vi "CMD_05_SetSendPeriod.vi"(9 "Period, ms":dbl=10.0 min=10.0 max=10000.0, 11 "VISA resource name":refnum<visa-resource-name>) -> (3 "VISA resource name out":refnum<visa-resource-name>)   [LabVIEW 2017]
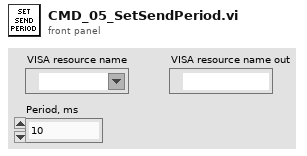
[diagram p1: front panel]
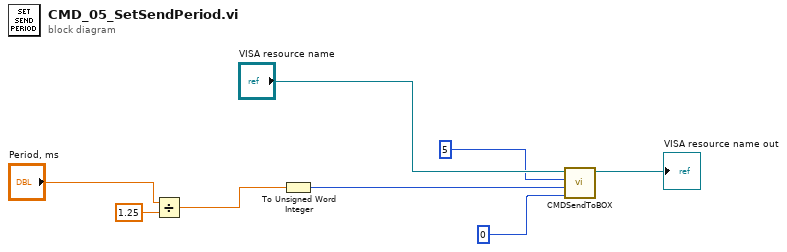
[diagram p0: block diagram]
diagram:
  n1 = Divide(x="Period, ms", y=1.25) -> (x/y=w2:dbl)
  n2 = To Unsigned Word Integer(number=w2) -> (unsigned 16bit integer=w3:u16)
  n3 = call "CMDSendToBOX.vi"("arg2"=i16 0, "arg1"=w3, "CMD"=i8 5, "VISA resource name"="VISA resource name") -> ("VISA resource name out"=→"VISA resource name out":refnum<visa-resource-name>)  [unwired: 7 in]
